vi "calc MOD COORDS.vi"(8 "error in (no error)":errorcluster) -> (0 "error out":errorcluster, 3 "CG info":T2={"mass (lbm)"=150.0, "Xcg"=24.0, "Ycg"=0.0, "Zcg"=24.0})   [LabVIEW 2023]
uses:
  ctrl defs/ctrl robot CG.ctl
  ctrl defs/ctrl swerve module.ctl
  Global INIT.vi
  Global odometry.vi
panel:
  out "SWERVE INFO":T1[](array[typedef]) {"corner wt (lbm)" format="%.4g"; "angle" format="%.3g"; "coord wrt geom CTR"."geomY" format="%.4g"; "coord wrt geom CTR"."geomX" format="%.4g"; "from CG to module"."theta cg (deg)" format="%.4g"; "from CG to module"."Rcg" format="%.4g"; "POS delta" format="%.3g"; "POS last" format="%.3g"; "POS target" format="%.3g"; "V" format="%.3g"}
  out "coord wrt geom ctr":cluster{"X":dbl, "Y":dbl}[](array[cluster])
  out "CG XY":cluster{"X":dbl, "Y":dbl}
  out "wheel track & base":cluster{"X":dbl, "Y":dbl}={"X"=24.428, "Y"=24.428}
  out "weight (lbm)":dbl
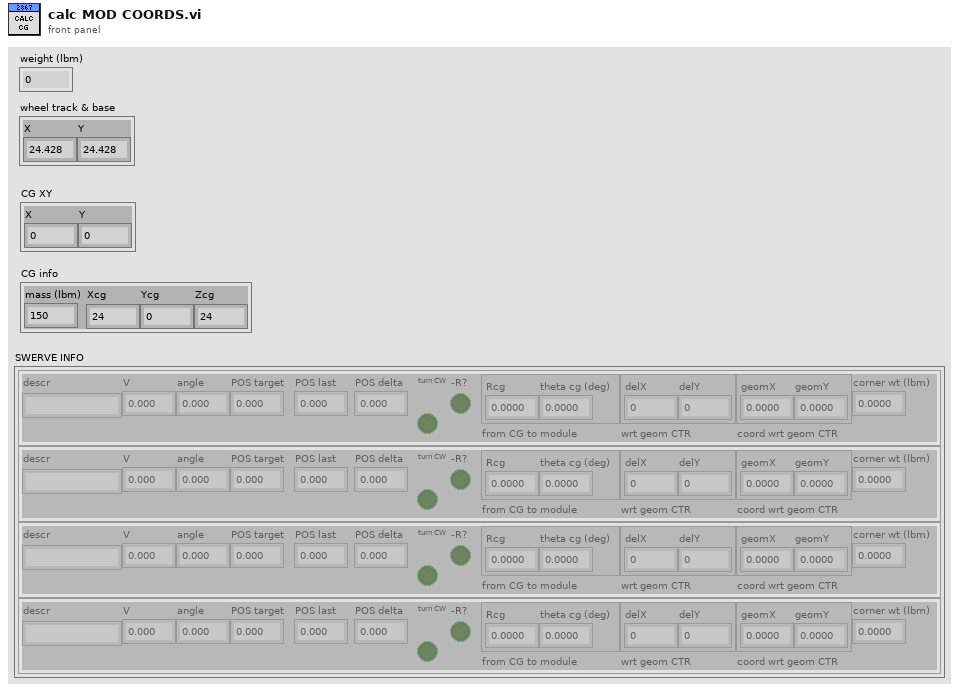
[diagram p1: front panel]
types:
  T1 = typedef "ctrl swerve module.ctl" = cluster{"descr":string, "V":dbl, "angle":dbl, "POS target":dbl, "POS last":dbl, "POS delta":dbl, "turn CW":bool, "-R?":bool, "from CG to module":cluster{"Rcg":dbl, "theta cg (deg)":dbl}, "wrt geom CTR":cluster{"delX":i8, "delY":i8}, "coord wrt geom CTR":cluster{"geomX":dbl, "geomY":dbl}, "corner wt (lbm)":dbl}
  T2 = typedef "ctrl robot CG.ctl" = cluster{"mass (lbm)":dbl, "Xcg":dbl, "Ycg":dbl, "Zcg":dbl}
  T3 = typedef "ctrl robot swerve dims.ctl" = cluster{"drive track":dbl, "drive base":dbl, "wheel  (in)":dbl, "steer ratio":dbl, "drive ratio":dbl, "enc ratio":dbl}
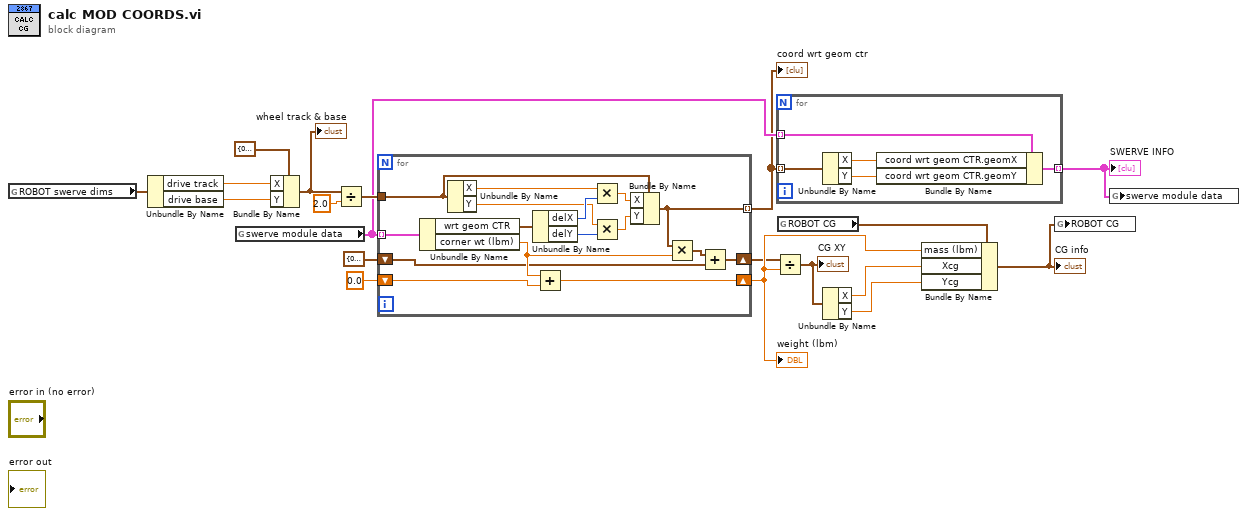
[diagram p0: block diagram]
diagram:
  n1 = global read "Global INIT.vi" "ROBOT swerve dims"() -> (w9:T3)
  n2 = Unbundle By Name(w9) -> ("drive track"=w14:dbl, "drive base"=w13:dbl)
  n3 = global read "Global odometry.vi" "swerve module data"() -> (w3:T1[])
  n4 = Bundle By Name(cluster=cluster{"X":dbl, "Y":dbl} {"X"=0.0, "Y"=0.0}, "X"=w14, "Y"=w13) -> (w12:cluster{"X":dbl, "Y":dbl})
  "wheel track & base" <- w12
  n5 = Divide(x=w12, y=2.0) -> (x/y=w8:cluster{"X":dbl, "Y":dbl})
  n6 = for {
    tunnel: w8 -> [w35]
    tunnel: [w25] -> w1 mode=indexing
    tunnel: w3 -> [w32] mode=indexing
    shift-right: [w24] -> w6
    shift-left: 0.0 -> [w31]
    shift-right: [w21] -> w4
    shift-left: cluster{"X":dbl, "Y":dbl} {"X"=0.0, "Y"=0.0} -> [w20]
    n7 = Unbundle By Name(w32) -> ("wrt geom CTR"=w30:cluster{"delX":i8, "delY":i8}, "corner wt (lbm)"=w23:dbl)
    n8 = Unbundle By Name(w35) -> ("X"=w33:dbl, "Y"=w27:dbl)
    n9 = Unbundle By Name(w30) -> ("delX"=w29:i8, "delY"=w26:i8)
    n10 = Add(x=w23, y=w31) -> (x+y=w24:dbl)
    n11 = Multiply(x=w33, y=w29) -> (x*y=w34:dbl)
    n12 = Multiply(x=w27, y=w26) -> (x*y=w28:dbl)
    n13 = Bundle By Name(cluster=w35, "X"=w34, "Y"=w28) -> (w25:cluster{"X":dbl, "Y":dbl})
    n14 = Multiply(x=w25, y=w23) -> (x*y=w22:cluster{"X":dbl, "Y":dbl})
    n15 = Add(x=w22, y=w20) -> (x+y=w21:cluster{"X":dbl, "Y":dbl})
  }
  "weight (lbm)" <- w6
  "coord wrt geom ctr" <- w1
  n16 = Divide(x=w4, y=w6) -> (x/y=w17:cluster{"X":dbl, "Y":dbl})
  "CG XY" <- w17
  n17 = for {
    tunnel: w3 -> [w40] mode=indexing
    tunnel: [w39] -> w2 mode=indexing
    tunnel: w1 -> [w38] mode=indexing
    n18 = Unbundle By Name(w38) -> ("X"=w37:dbl, "Y"=w36:dbl)
    n19 = Bundle By Name(cluster=w40, "coord wrt geom CTR.geomX"=w37, "coord wrt geom CTR.geomY"=w36) -> (w39:T1)
  }
  "SWERVE INFO" <- w2
  n20 = global read "Global INIT.vi" "ROBOT CG"() -> (w19:T2)
  n21 = Unbundle By Name(w17) -> ("X"=w16:dbl, "Y"=w15:dbl)
  n22 = Bundle By Name(cluster=w19, "mass (lbm)"=w6, "Xcg"=w16, "Ycg"=w15) -> (w18:T2)
  "CG info" <- w18
  n23 = global write "Global INIT.vi" "ROBOT CG"(w18) -> ()
  n24 = global write "Global odometry.vi" "swerve module data"(w2) -> ()
